vi "MsgBox_Win.vi"(8 "Error in":errorcluster caption="Error in (no error)", 9 "timeout (ms)":i32=3000, 10 "strCaption":string, 11 "strText":string) -> (0 "Error out":errorcluster, 3 "Return Value":u32)   [LabVIEW 2013]
uses:
  Windows/System32/user32.dll
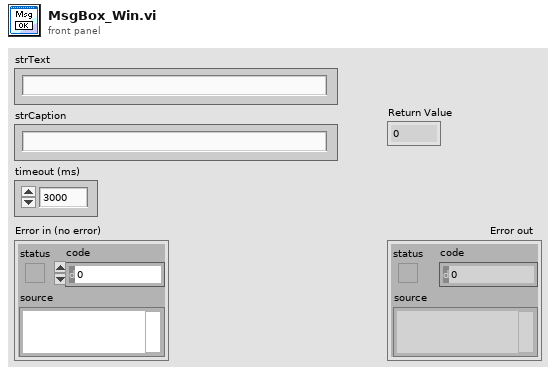
[diagram p1: front panel]
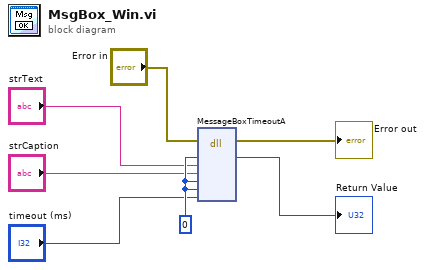
[diagram p0: block diagram]
diagram:
  w5 = 0 ("NULL")
  n1 = dll-call lib="C:/Windows/System32/user32.dll" fn="MessageBoxTimeoutA" label="MessageBoxTimeout"(error in="Error in", "NULL"=w5, "strText"="strText", "strCaption"="strCaption", "MB_OK"=w5, "0"=w5, "sec*1000"="timeout (ms)") -> (error out=→"Error out":errorcluster, "NULL"=→"Return Value":i32)  [unwired: 8 in, 1 out]
